vi "solar_misc LVClass Hierarchy.vi"(8 "error in (no error)":errorcluster) -> (0 "error out":errorcluster, 2 "LVClass Hierarchy":cluster{"Inheritance":string[]}[](array[cluster]), 3 "All LVClasses in Memory":string[](array[string]))   [LabVIEW 2018]
doc: "This VI gets the LabVIEW Class Hierarchy of all classes loaded in memory.\n\nCreated By: Ryan Pacini\nDate: 5/28/2016"
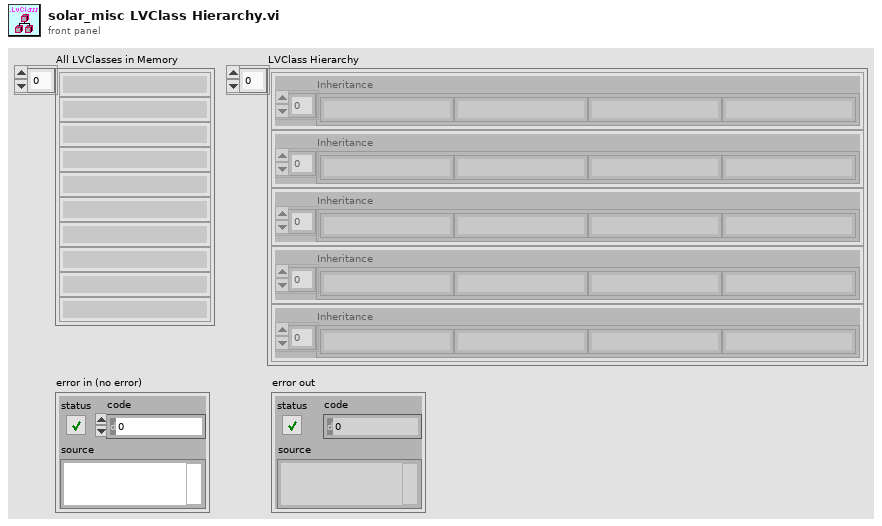
[diagram p1: front panel]
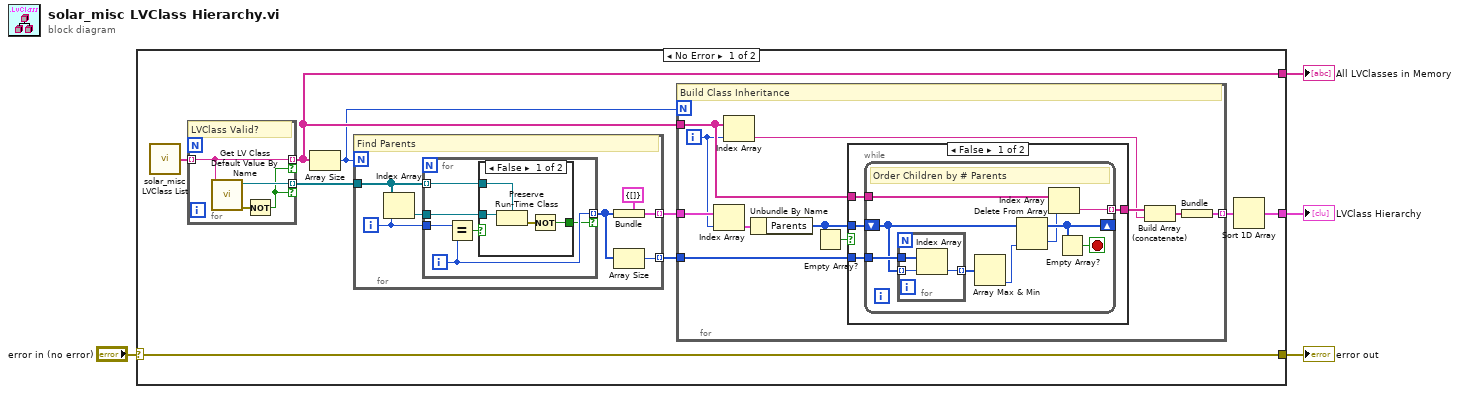
[diagram p0: block diagram]
diagram:
  n1 = case shown="No Error" "error in (no error)" {
    selector: "error in (no error)" -> [w5 w62]
    tunnel: [w13 _] -> w4
    tunnel: [w12 _] -> w3
    tunnel: [w5 w62] -> w2
    frame No Error {
      n2 = call "solar_misc LVClass List.vi"() -> ("All LVClasses in Memory"=w6:string[])
      n3 = for {
        tunnel: w6 -> [w60] mode=indexing
        tunnel: [w61] -> w7 mode=indexing if=w58
        tunnel: [w60] -> w13 mode=indexing if=w58
        # "LVClass Valid?"
        n4 = call <vilib>:"Get LV Class Default Value By Name.vi"("class name"=w60) -> ("error out"=w59:errorcluster, "object"=w61:refnum<class>)  [unwired: 9 in]
        n5 = Not(x=w59) -> (.not. x?=w58:bool)
      }
      n6 = Array Size(array=w13) -> (size(s)=w11:i32)
      n7 = for {
        N: w11 -> [_]
        tunnel: w7 -> [w41]
        tunnel: [w47] -> w8 mode=indexing
        tunnel: [w43] -> w10 mode=indexing
        i -> [w45]
        # "Find Parents"
        n8 = Index Array(array=w41, index=w45) -> (element=w46:refnum<class>)
        n9 = for {
          tunnel: w46 -> [w53]
          tunnel: w41 -> [w52] mode=indexing
          tunnel: [w51] -> w42 mode=indexing if=w49
          tunnel: w45 -> [w50]
          i -> [w51]
          n10 = Equal?(x=w50, y=w51) -> (x = y?=w48:bool)
          n11 = case shown="False" w48 {
            tunnel: w53 -> [w57 _]
            tunnel: w52 -> [w56 _]
            tunnel: [w54 _] -> w49
            frame False {
              n12 = Preserve Run-Time Class(object in=w57, 2:w56) -> (error out=w55:errorcluster)  [unwired: 1 in, 1 out]
              n13 = Not(x=w55) -> (.not. x?=w54:bool)
            }
            frame True {
              # "Ignore\nSelf"
            }
          }
        }
        n14 = Bundle(cluster=cluster{"Parents":i32[]} {"Parents"=[]} ("Inheritance"), "Parents"=w42) -> (w47:cluster{"Parents":i32[]})
        n15 = Array Size(array=w42) -> (size(s)=w43:i32)
      }
      n16 = for {
        N: w11 -> [_]
        tunnel: w8 -> [w22]
        tunnel: w10 -> [w23]
        tunnel: [w20] -> w9 mode=indexing
        tunnel: w13 -> [w15]
        i -> [w14]
        # "Build Class Inheritance"
        n17 = Index Array(array=w22, index=w14) -> (element=w21:cluster{"Parents":i32[]})
        n18 = Index Array(array=w15, index=w14) -> (element=w16:string)
        n19 = Unbundle By Name(w21) -> ("Parents"=w19:i32[])
        n20 = Empty Array?(array=w19) -> (empty?=w17:bool)
        n21 = case shown="False" w17 {
          tunnel: w23 -> [w28 _]
          tunnel: w15 -> [w27 _]
          tunnel: w19 -> [w26 _]
          tunnel: [w25 _] -> w18
          frame False {
            n22 = while {
              tunnel: w28 -> [w37]
              tunnel: w27 -> [w31]
              shift-right: [w34] -> _
              shift-left: w26 -> [w35]
              tunnel: [w29] -> w25 mode=indexing
              stop <- w33 stop-if-true
              # "Order Children by # Parents"
              n23 = for {
                tunnel: w37 -> [w40]
                tunnel: w35 -> [w39] mode=indexing
                tunnel: [w38] -> w36 mode=indexing
                n24 = Index Array(array=w40, index=w39) -> (element=w38:i32)
              }
              n25 = Array Max & Min(array=w36) -> (min index (indices)=w32:i32)  [unwired: 3 out]
              n26 = Delete From Array(array=w35, index=w32) -> (deleted portion=w30:i32, array with subset deleted=w34:i32[])  [unwired: 1 in]
              n27 = Index Array(array=w31, index=w30) -> (element=w29:string)
              n28 = Empty Array?(array=w34) -> (empty?=w33:bool)
            }
          }
          frame True {
          }
        }
        n29 = Build Array (concatenate)(w18, w16) -> (w24:string[])
        n30 = Bundle(w24) -> (w20:cluster{string[]})  [unwired: 1 in]
      }
      n31 = Sort 1D Array(array=w9) -> (sorted array=w12:cluster{string[]}[])
    }
    frame Error {
    }
  }
  "All LVClasses in Memory" <- w4
  "LVClass Hierarchy" <- w3
  "error out" <- w2
